vi "JSON-GlobalParseDB.vi"(10 "error in (no error)":errorcluster, 11 "Payload From DB Actor":string) -> (2 "error out":errorcluster, 5 "columns":string[](array[string]), 7 "data":string[][](array[string]))   [LabVIEW 2014]
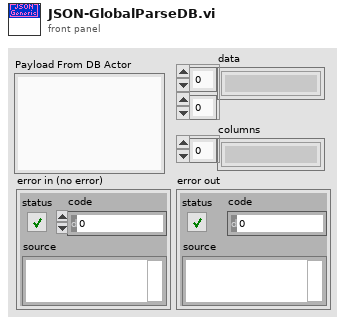
[diagram p1: front panel]
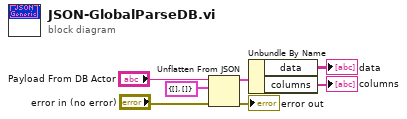
[diagram p0: block diagram]
diagram:
  n1 = Unflatten From JSON(JSON string="Payload From DB Actor", type and defaults=cluster{"data":string[][], "columns":string[]} {"data"=[], "columns"=[]}, error in (no error)="error in (no error)") -> (value=w7:cluster{"data":string[][], "columns":string[]}, error out=→"error out":errorcluster)  [unwired: 4 in]
  n2 = Unbundle By Name(w7) -> ("data"=→"data":string[][], "columns"=→"columns":string[])
